vi "MovePilMot.vi"(0 "Ordre UC":u16=1, 1 "Variables d'Axes":T2={"OrdreBloc"="ni.var.psp://localhost/OPC/OPC1/esbimETH_1/module1/2AXBOC/E0_Ordre/Axe2_OrdreBloc", "Ordre UC"="ni.var.psp://localhost/OPC/OPC1/esbimETH_1/module1/2AXBOC/E0_Ordre/Axe2_OrdreUC", "CoteAAtteindre"="ni.var.psp://localhost/OPC/OPC1/esbimETH_1/module1/2AXBOC/E2_Position2/CoteAAtteindre", "Vitesse"="ni.var.psp://localhost/OPC/OPC1/esbimETH_1/module1/2AXBOC/E2_Position2/Vitesse", "Position codeur en pas"="ni.var.psp://localhost/OPC/OPC1/esbimETH_1/module1/2AXBOC/L4_PositionPas/Axe2_PositionCodeurEnPas", "Position Théorique"="ni.var.psp://localhost/OPC/OPC1/esbimETH_1/module1/2AXBOC/L0_Position/Axe2_PositionTheorique", "Message"="ni.var.psp://localhost/OPC/OPC1/esbimETH_1/module1/2AXBOC/L0_Position/Axe2_Messages", "Ecrire"="ni.var.psp://localhost/OPC/OPC1/esbimETH_1/module1/2AXBOC/ecrire", "Zone à écrire"="ni.var.psp://localhost/OPC/OPC1/esbimETH_1/module1/2AXBOC/zones_a_ecrire", "Numéro paramètre"="ni.var.psp://localhost/OPC/OPC1/esbimETH_1/module1/2AXBOC/E3_Parametres/NumeroParametre", "Ordre"="ni.var.psp://localhost/OPC/OPC1/esbimETH_1/module1/2AXBOC/E3_Parametres/Ordre", "Valeur"="ni.var.psp://localhost/OPC/OPC1/esbimETH_1/module1/2AXBOC/E3_Parametres/Valeur", "Valeur Lecture"="ni.var.psp://localhost/OPC/OPC1/esbimETH_1/module1/2AXBOC/L2_Parametres/Valeur", "Numéro paramètre Lecture"="ni.var.psp://localhost/OPC/OPC1/esbimETH_1/module1/2AXBOC/L2_Parametres/Numero", "Acquittement Lecture Ecriture"="ni.var.psp://localhost/OPC/OPC1/esbimETH_1/module1/2AXBOC/L2_Parametres/AcquitementLectureEcriture", "Zone à Ecrire Pour Axe "=0, "Acquittement Ordre UC"=""}, 5 "Cote à atteindre":i32, 9 "Vitesse":i32=1000, 11 "error in (no error)":errorcluster caption="entrée d'erreur (pas d'erreur)", 12 "Type de mouvement":T1=2 items=["Mouvement Simple"=1, "Aller vers Cote"=2, "Va vers position de référence"=3], 13 "Mouvement Absolu/Relatif":u16(ring) items=["Mouvement Relatif"=1, "Mouvement Absolu"=0], 14 "Ordre Bloc":u16=1) -> (15 "error out":errorcluster caption="sortie d'erreur")   [LabVIEW 2014]
uses:
  AdressesVariablesPartagees.ctl
  Commandes/Type de Mouvement PilMOT.ctl
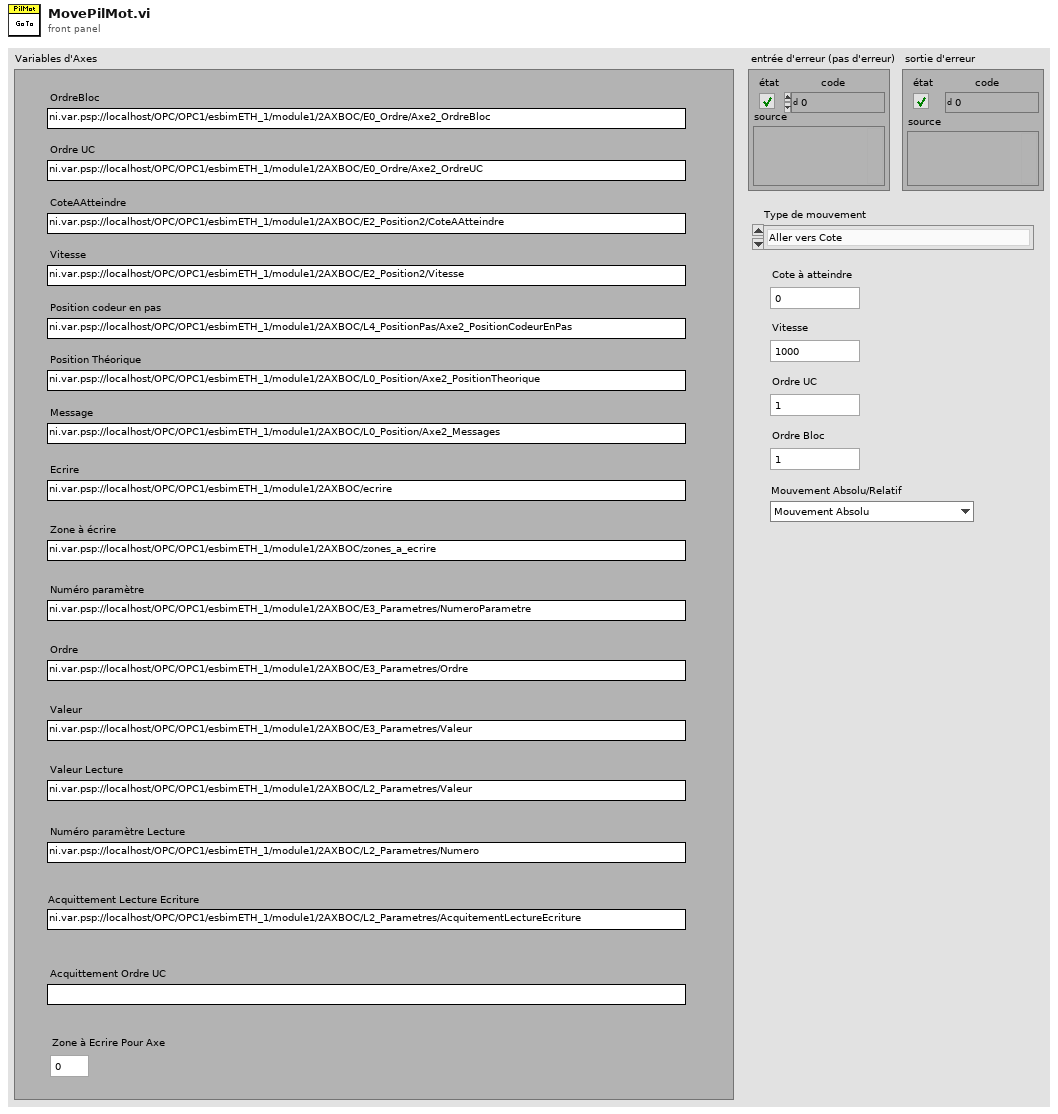
[diagram p1: front panel]
types:
  T1 = typedef "Type de Mouvement PilMOT.ctl" = u16
  T2 = typedef "AdressesVariablesPartagees.ctl" = cluster{"OrdreBloc":string, "Ordre UC":string, "CoteAAtteindre":string, "Vitesse":string, "Position codeur en pas":string, "Position Théorique":string, "Message":string, "Ecrire":string, "Zone à écrire":string, "Numéro paramètre":string, "Ordre":string, "Valeur":string, "Valeur Lecture":string, "Numéro paramètre Lecture":string, "Acquittement Lecture Ecriture":string, "Zone à Ecrire Pour Axe ":u16, "Acquittement Ordre UC":string}
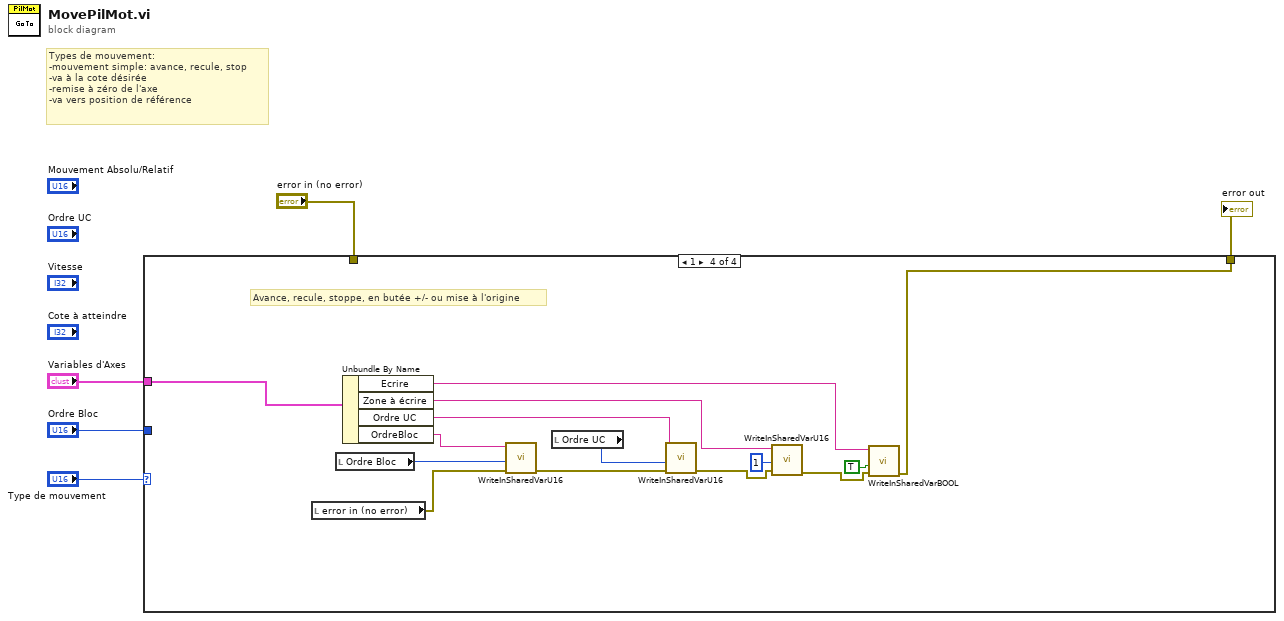
[diagram p0: block diagram]
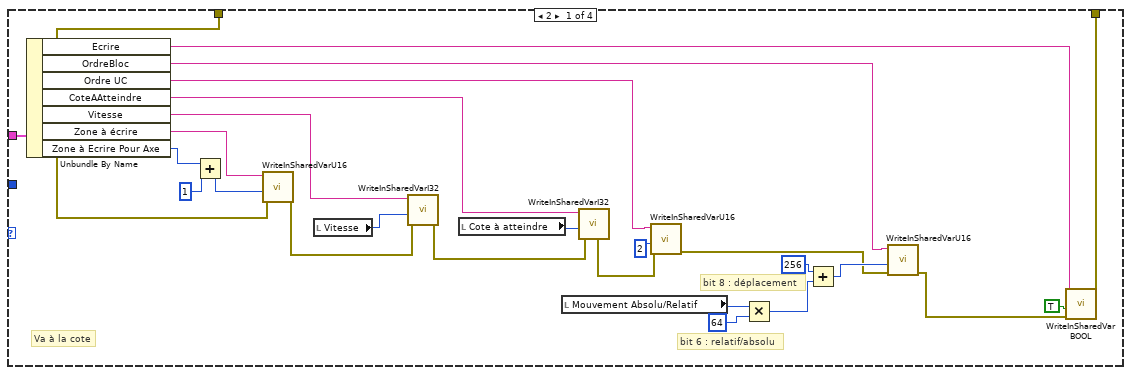
[diagram p2: hidden frame]
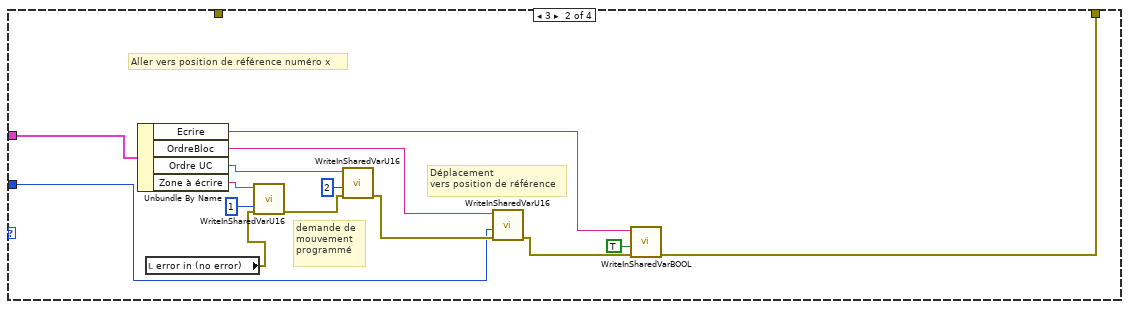
[diagram p3: hidden frame]
diagram:
  # "Types de mouvement:\n-mouvement simple: avance, recule, stop\n-va à la cote désirée\n-remise à zéro de l'axe\n-va vers position de référence"
  n1 = case shown="1" "Type de mouvement" {
    tunnel: "Variables d'Axes" -> [w31 w45 _ w60]
    tunnel: [w29 w37 w46 w47] -> w5
    tunnel: "error in (no error)" -> [w24 _ w46 _]
    tunnel: "Ordre Bloc" -> [_ w32 _ _]
    frame 2 {
      # "bit 6 : relatif/absolu"
      # "bit 8 : déplacement"
      # "Va à la cote"
      n2 = Unbundle By Name(w31) -> ("Ecrire"=w22:string, "OrdreBloc"=w7:string, "Ordre UC"=w14:string, "CoteAAtteindre"=w17:string, "Vitesse"=w20:string, "Zone à écrire"=w23:string, "Zone à Ecrire Pour Axe"=w26:u16)
      n3 = Add(x=w26, y=u16 1 ("données en entrée")) -> (x+y=w25:u16)
      n4 = call "WriteInSharedVarU16.vi"("entrée d'erreur (pas d'erreur)"=w24, "données en entrée"=w25, "refnum de variable partagée en entrée"=w23) -> ("sortie d'erreur"=w28:errorcluster)  [unwired: 8 in]
      n5 = local read "Vitesse"() -> (w21:i32)
      n6 = call "WriteInSharedVarI32.vi"("entrée d'erreur (pas d'erreur)"=w28, "données en entrée"=w21, "refnum de variable partagée en entrée"=w20) -> ("sortie d'erreur"=w18:errorcluster)  [unwired: 8 in]
      n7 = local read "Cote à atteindre"() -> (w19:i32)
      n8 = local read "Mouvement Absolu/Relatif"() -> (w13:u16)
      n9 = call "WriteInSharedVarI32.vi"("entrée d'erreur (pas d'erreur)"=w18, "données en entrée"=w19, "refnum de variable partagée en entrée"=w17) -> ("sortie d'erreur"=w15:errorcluster)  [unwired: 8 in]
      n10 = call "WriteInSharedVarU16.vi"("entrée d'erreur (pas d'erreur)"=w15, "données en entrée"=u16 2, "refnum de variable partagée en entrée"=w14) -> ("sortie d'erreur"=w8:errorcluster)  [unwired: 8 in]
      n11 = Multiply(x=w13, y=u16 64) -> (x*y=w10:u16)
      n12 = Add(x=u16 256 ("données en entrée"), y=w10) -> (x+y=w9:u16)
      n13 = call "WriteInSharedVarU16.vi"("entrée d'erreur (pas d'erreur)"=w8, "données en entrée"=w9, "refnum de variable partagée en entrée"=w7) -> ("sortie d'erreur"=w6:errorcluster)  [unwired: 8 in]
      n14 = call "WriteInSharedVarBOOL.vi"("entrée d'erreur (pas d'erreur)"=w6, "données en entrée"=TRUE, "refnum de variable partagée en entrée"=w22) -> ("sortie d'erreur"=w29:errorcluster)  [unwired: 8 in]
    }
    frame 3 {
      # "Déplacement\nvers position de référence"
      # "demande de\nmouvement \nprogrammé"
      # "Aller vers position de référence numéro x"
      n15 = Unbundle By Name(w45) -> ("Ecrire"=w41:string, "OrdreBloc"=w42:string, "Ordre UC"=w36:string, "Zone à écrire"=w44:string)
      n16 = local read "error in (no error)"() -> (w38:errorcluster)
      n17 = call "WriteInSharedVarU16.vi"("entrée d'erreur (pas d'erreur)"=w38, "données en entrée"=u16 1, "refnum de variable partagée en entrée"=w44) -> ("sortie d'erreur"=w34:errorcluster)  [unwired: 8 in]
      n18 = call "WriteInSharedVarU16.vi"("entrée d'erreur (pas d'erreur)"=w34, "données en entrée"=u16 2, "refnum de variable partagée en entrée"=w36) -> ("sortie d'erreur"=w33:errorcluster)  [unwired: 8 in]
      n19 = call "WriteInSharedVarU16.vi"("entrée d'erreur (pas d'erreur)"=w33, "données en entrée"=w32, "refnum de variable partagée en entrée"=w42) -> ("sortie d'erreur"=w43:errorcluster)  [unwired: 8 in]
      n20 = call "WriteInSharedVarBOOL.vi"("entrée d'erreur (pas d'erreur)"=w43, "données en entrée"=TRUE, "refnum de variable partagée en entrée"=w41) -> ("sortie d'erreur"=w37:errorcluster)  [unwired: 8 in]
    }
    frame 0, Default {
    }
    frame 1 {
      # "Avance, recule, stoppe, en butée +/- ou mise à l'origine"
      n21 = local read "error in (no error)"() -> (w50:errorcluster)
      n22 = local read "Ordre Bloc"() -> (w48:u16)
      n23 = Unbundle By Name(w60) -> ("Ecrire"=w55:string, "Zone à écrire"=w57:string, "Ordre UC"=w59:string, "OrdreBloc"=w49:string)
      n24 = call "WriteInSharedVarU16.vi"("entrée d'erreur (pas d'erreur)"=w50, "données en entrée"=w48, "refnum de variable partagée en entrée"=w49) -> ("sortie d'erreur"=w51:errorcluster)  [unwired: 8 in]
      n25 = local read "Ordre UC"() -> (w53:u16)
      n26 = call "WriteInSharedVarU16.vi"("entrée d'erreur (pas d'erreur)"=w51, "données en entrée"=w53, "refnum de variable partagée en entrée"=w59) -> ("sortie d'erreur"=w58:errorcluster)  [unwired: 8 in]
      n27 = call "WriteInSharedVarU16.vi"("entrée d'erreur (pas d'erreur)"=w58, "données en entrée"=u16 1, "refnum de variable partagée en entrée"=w57) -> ("sortie d'erreur"=w54:errorcluster)  [unwired: 8 in]
      n28 = call "WriteInSharedVarBOOL.vi"("entrée d'erreur (pas d'erreur)"=w54, "données en entrée"=TRUE, "refnum de variable partagée en entrée"=w55) -> ("sortie d'erreur"=w47:errorcluster)  [unwired: 8 in]
    }
  }
  "error out" <- w5
